vi "arduinotalker.vi"() -> ()   [LabVIEW 2021]
uses:
  <vilib>/Instr/_visa.llb/VISA Configure Serial Port (Instr).vi
panel:
  out "resulting string":string
  in  "Slide":dbl(slide) scale=0.0..255.0
  in  "VISA resource name":refnum<visa-resource-name>
  in  "stop":bool
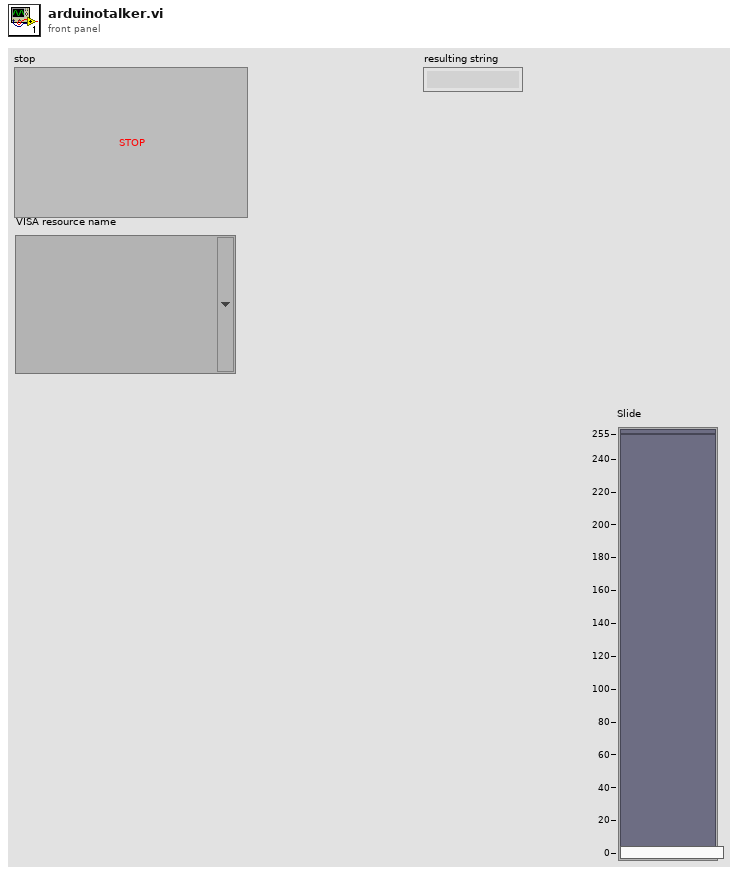
[diagram p1: front panel]
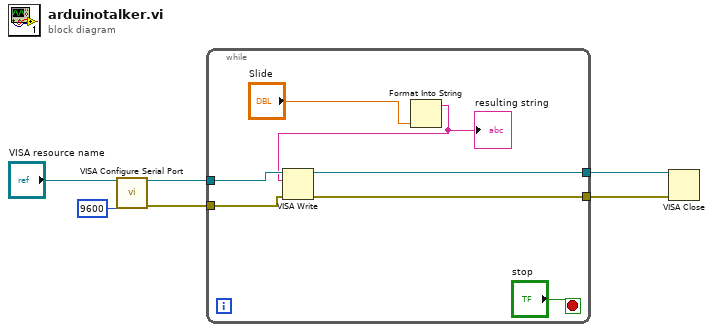
[diagram p0: block diagram]
diagram:
  n1 = call-poly "VISA Configure Serial Port"("VISA resource name"="VISA resource name", "baud rate (9600)"=u32 9600) -> ("VISA resource name out"=w4:refnum<visa-resource-name>, "error out"=w2:errorcluster)  [unwired: 12 in]
  n2 = while {
    tunnel: w4 -> [w12]
    tunnel: [w11] -> w3
    tunnel: w2 -> [w10]
    tunnel: [w9] -> w1
    stop <- "stop" stop-if-true
    n3 = Format Into String("Slide") -> (resulting string=w7:string)  [unwired: 3 in, 1 out]
    "resulting string" <- w7
    n4 = VISA Write(VISA resource name=w12, write buffer=w7, error in (no error)=w10) -> (VISA resource name out=w11:refnum<visa-resource-name>, error out=w9:errorcluster)  [unwired: 1 out]
  }
  n5 = VISA Close(VISA resource name=w3, error in (no error)=w1) -> ()  [unwired: 1 out]
